vi "Power-HWP test.vi"(8 "Error In":errorcluster, 10 "Cluster In":T1={"Position"=0.0, "Is.Enabled?"=FALSE, "Is.Connected?"=FALSE, "Device SN"="55151324", "AccelerationMaximum"=10.0, "VelocityMaximum"=10.0, "Acceleration"=10.0, "Velocity"=10.0, "waitTimeout (ms)"=10000, "Model"=enum."None", "Is.Homed?"=FALSE}) -> (0 "Error Out":errorcluster)   [LabVIEW 2018]
uses:
  Hardware Mfg/Thorlabs Translation Stages/Controls/Translation Stage Cluster.ctl
  General/Controls/Translation Stage Types.ctl
  KnifeEdgeTestClt.ctl
  Hardware Mfg/Thorlabs Cage Rotation/refnum control.ctl
  General/Controls/Set Get Controls.ctl
  Hardware Mfg/Thorlabs Translation Stages/Controls/Motion Translation Module Control2.ctl
  C:/Project/SerialSectionOCT/SerialSectOCT/Labview Software/Thorlabs.MotionControl.Controls.dll
  Thorlabs.MotionControl.Controls.dll
panel:
  in  "LTS Reference":refnum<k24>(container)
  out "Power":dbl
  in  "Start":dbl
  in  "Stop":dbl
  in  "step size":dbl
  out "Wavelength [nm] 2":dbl caption="Wavelength"
  out "Avg. Time  [sec.]":dbl caption="Average Time"
  out "Average Count 2":i32 caption="Average Time"
  in  "Avg. Time (0.0) [sec.]":dbl=1.5 caption="Average Time (0.0)" min=0.1 max=5.0 step=0.1
  in  "Wavelength [nm]":dbl=840.0 caption="Wavelength (0.0)"
  in  "Average Count":i32=10 min=1 step=1
  in  "path":path=path "D:/200806 KnifeEdgeMeasurement"
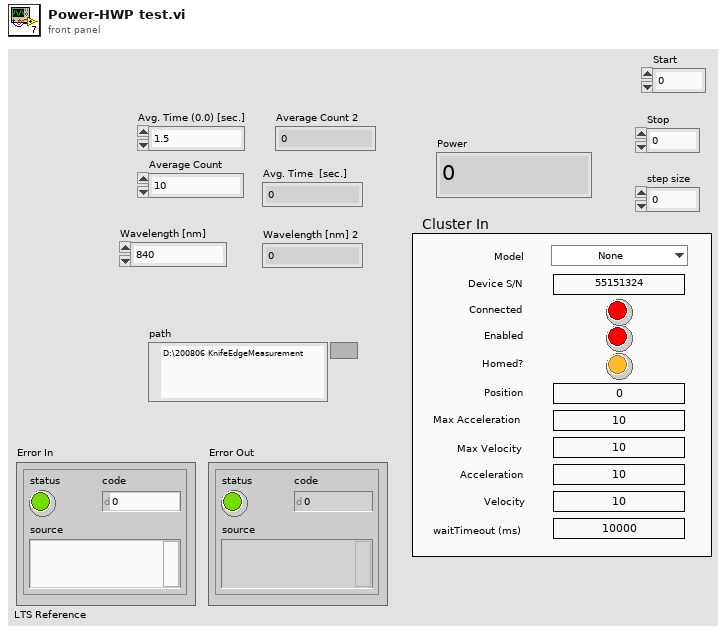
[diagram p1: front panel]
types:
  T1 = typedef "Translation Stage Cluster.ctl" = cluster{"Position":dbl, "Is.Enabled?":bool, "Is.Connected?":bool, "Device SN":string, "AccelerationMaximum":dbl, "VelocityMaximum":dbl, "Acceleration":dbl, "Velocity":dbl, "waitTimeout (ms)":i32, "Model":T2, "Is.Homed?":bool}
  T2 = typedef "Translation Stage Types.ctl" = enum16{"None", "Thorlabs LTS", "Thorlabs MLJ"}
  T3 = typedef "KnifeEdgeTestClt.ctl" = enum16{"Init Power meter", "Init Table stages", "Go stage home", "Move stage", "Measure power", "Uninit", "Generate steps"}
  T4 = typedef "refnum control.ctl" = enum16{"Get", "Init"}
  T5 = typedef "Motion Translation Module Control2.ctl" = enum16{"Init", "Home", "Status", "Velocity/Accel", "Position", "Jog", "Stop", "Uninit", "Enable", "Disable"}
  T6 = typedef "Set Get Controls.ctl" = enum16{"Set", "Get"}
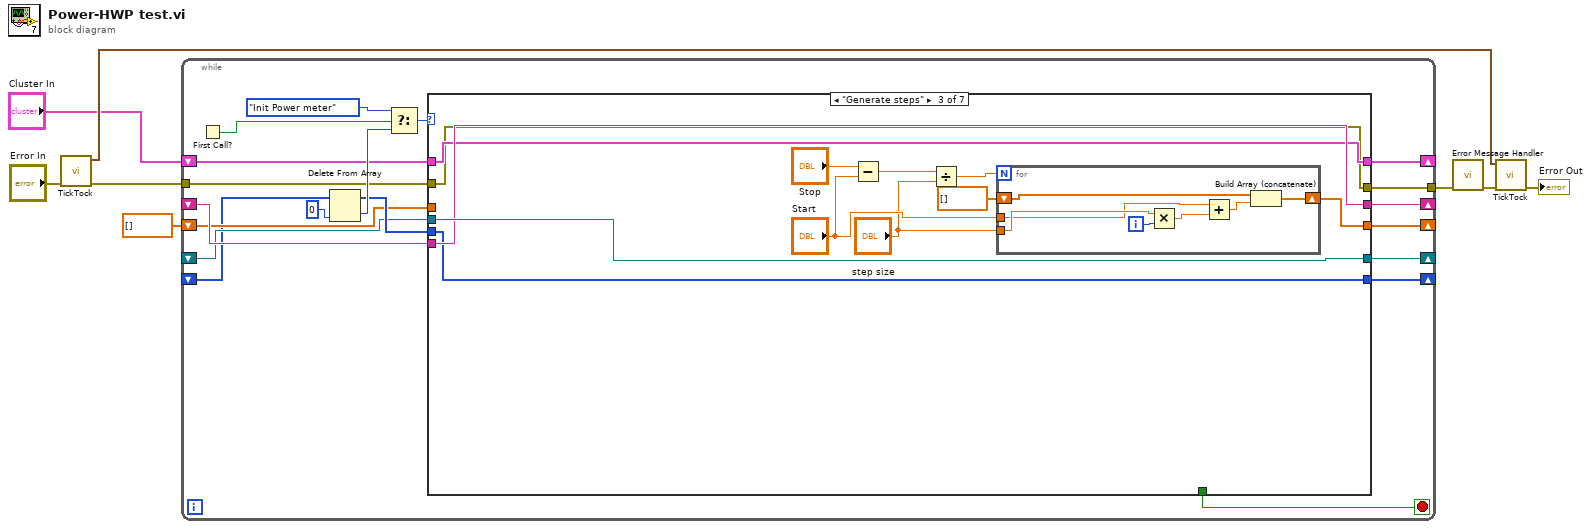
[diagram p0: block diagram]
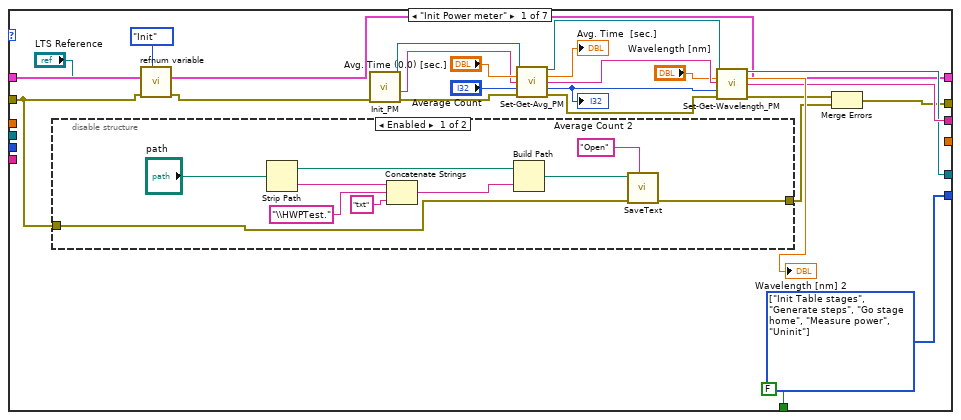
[diagram p2: hidden frame]
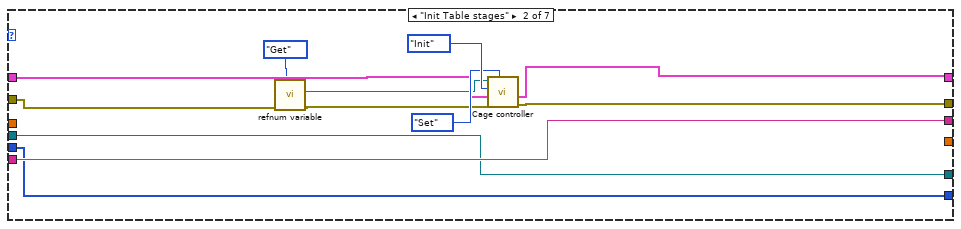
[diagram p4: hidden frame]
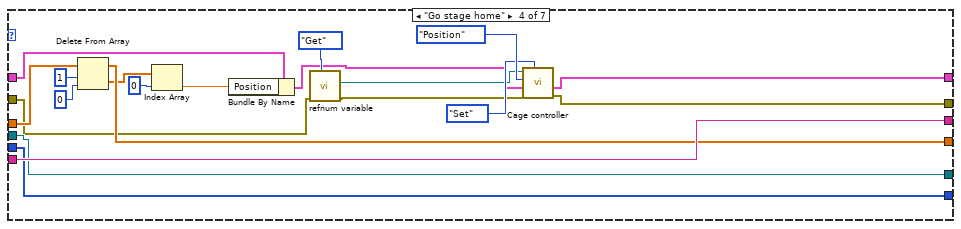
[diagram p5: hidden frame]
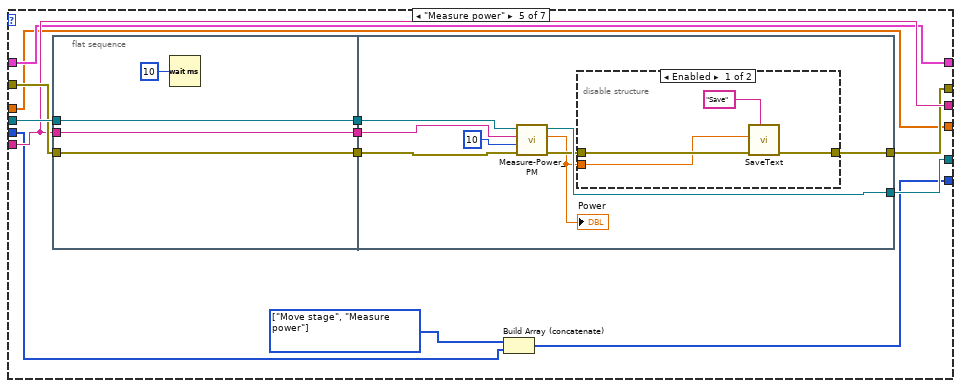
[diagram p6: hidden frame]
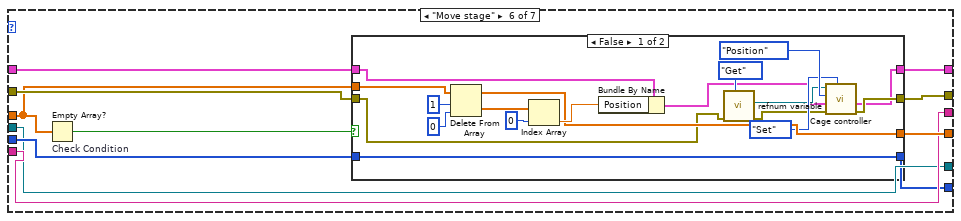
[diagram p8: hidden frame]
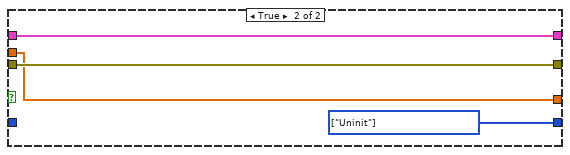
[diagram p9: hidden frame]
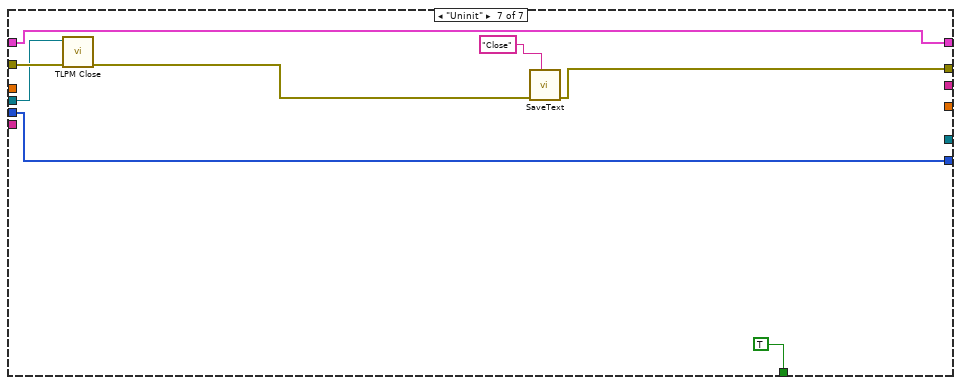
[diagram p10: hidden frame]
diagram:
  n1 = call "TickTock.vi"("Error In"="Error In") -> ("Error Out"=w6:errorcluster, "Current Time (Out)"=w4:timestamp)  [unwired: 8 in, 1 out]
  n2 = while {
    tunnel: w6 -> [w23]
    tunnel: [w22] -> w8
    shift-right: [w21] -> _
    shift-left: _ -> [w19]
    shift-right: [w20] -> _
    shift-left: _ -> [w18]
    shift-right: [w15] -> _
    shift-left: "Cluster In" -> [w16]
    shift-right: [w14] -> _
    shift-left: dbl[] [] -> [w13]
    shift-right: [w12] -> _
    shift-left: _ -> [w11]
    stop <- w10 stop-if-true
    n3 = First Call?() -> (First Call?: T/F=w9:bool)
    n4 = Delete From Array(array=w11, index=0) -> (deleted portion=w26:T3, array with subset deleted=w25:T3[])  [unwired: 1 in]
    n5 = Select(t=KnifeEdgeTestClt."Init Power meter", s=w9, f=w26) -> (s? t:f=w27:T3)
    n6 = case shown="\"Generate steps\"" w27 {
      tunnel: [w34 w71 w75 w103 w113 w144 w181] -> w12
      tunnel: w25 -> [_ w71 w75 w103 w114 w151 w181]
      tunnel: [_ _ w76 w108 w116 w153 _] -> w14
      tunnel: w23 -> [w31 w64 w82 w96 w124 w150 w183]
      tunnel: [w36 w70 w82 w95 w121 w149 w177] -> w22
      tunnel: [w39 w73 w84 w112 w122 w148 _] -> w21
      tunnel: [w38 w72 w85 w102 w123 w147 _] -> w20
      tunnel: w19 -> [_ w73 w84 w112 w122 w148 _]
      tunnel: w18 -> [_ w72 w85 w102 w125 w147 w182]
      tunnel: w16 -> [w33 w67 w83 w107 w117 w146 w180]
      tunnel: [w33 w66 w83 w93 w117 w145 w180] -> w15
      tunnel: w13 -> [_ _ _ w111 w116 w143 _]
      tunnel: [FALSE _ _ _ _ _ TRUE] -> w10
      frame "Init Power meter" {
        w34 = T3[] [enum."Init Table stages", enum."Generate steps", enum."Go stage home", enum."Measure power", enum."Uninit"] items=["Init Power meter", "Init Table stages", "Go stage home", "Move stage", "Measure power", "Uninit", "Generate steps"]
        n7 = disable-structure shown="Enabled" {
          disable-tunnel: w31 -> [w56 _]
          disable-tunnel: [w55 _] -> w37
          frame Enabled {
            n8 = Strip Path(path="path") -> (stripped path=w53:path, name=w59:string)
            n9 = Concatenate Strings(w59, "\\HWPTest." ("string"), "txt" ("string")) -> (w54:string)
            n10 = Build Path(base path=w53, name or relative path=w54) -> (appended path=w52:path)
            n11 = call "SaveText.vi"("action"="Open", "error in"=w56, "file path (use dialog)"=w52) -> ("error out"=w55:errorcluster)  [unwired: 8 in]
          }
          frame Disabled {
          }
        }
        n12 = call "refnum variable.vi"("action"=refnum_control."Init", "error in (no error)"=w31, "reference in"="LTS Reference") -> ("error out"=w30:errorcluster)  [unwired: 7 in, 1 out]
        n13 = call "Init_PM.vi"("error in (no error)"=w30) -> ("error out"=w40:errorcluster, "Sensor Name"=w41:string, "instrument handle out"=w42:refnum<visa-resource-name>)  [unwired: 8 in]
        n14 = call "Set-Get-Avg_PM.vi"("instrument handle"=w42, "Average Time (0.0)"="Avg. Time (0.0) [sec.]", "Sensor"=w41, "Average Count"="Average Count", "error in (no error)"=w40) -> ("instrument handle out"=w49:refnum<visa-resource-name>, "Average Time"=→"Avg. Time  [sec.]":dbl, "Sensor 2"=w47:string, "Average Count"=w46:i32, "error out"=w50:errorcluster)  [unwired: 6 in]
        "Average Count 2" <- w46
        n15 = call "Set-Get-Wavelength_PM.vi"("instrument handle"=w49, "Wavelength"="Wavelength [nm]", "Sensor Name"=w47, "Average Count"=w46, "error in (no error)"=w50) -> ("instrument handle out"=w38:refnum<visa-resource-name>, "Wavelength"=→"Wavelength [nm] 2":dbl, "Sensor Name 2"=w39:string, "error out"=w35:errorcluster)  [unwired: 6 in, 1 out]
        n16 = Merge Errors(w35, w37) -> (w36:errorcluster)
      }
      frame "Init Table stages" {
        n17 = call "refnum variable.vi"("action"=refnum_control."Get", "error in (no error)"=w64) -> ("error out"=w63:errorcluster, "reference in 2"=w62:refnum<k24>)  [unwired: 8 in]
        n18 = call "Cage controller.vi"("Set/Get"=Set_Get_Controls."Set", "error in (no error)"=w63, "Cluster In"=w67, "Action"=Motion_Translation_Module_Control2."Init", "reference in"=w62) -> ("error out"=w70:errorcluster, "Cluster out"=w66:T1)  [unwired: 4 in, 1 out]
      }
      frame "Generate steps" {
        n19 = Subtract(x="Stop", y="Start") -> (x-y=w80:dbl)
        n20 = Divide(x=w80, y="step size") -> (x/y=w79:dbl)
        n21 = for {
          N: w79 -> [_]
          tunnel: "Start" -> [w90]
          tunnel: "step size" -> [w91]
          shift-right: [w87] -> w76
          shift-left: dbl[] [] -> [w86]
          i -> [w92]
          n22 = Multiply(x=w91, y=w92) -> (x*y=w89:dbl)
          n23 = Add(x=w90, y=w89) -> (x+y=w88:dbl)
          n24 = Build Array (concatenate)(w86, w88) -> (w87:dbl[])
        }
      }
      frame "Go stage home" {
        n25 = Delete From Array(array=w111, length=1, index=0) -> (deleted portion=w106:dbl[], array with subset deleted=w108:dbl[])
        n26 = Index Array(array=w106, index=0) -> (element=w104:dbl)
        n27 = Bundle By Name(cluster=w107, "Position"=w104) -> (w94:T1)
        n28 = call "refnum variable.vi"("action"=refnum_control."Get", "error in (no error)"=w96) -> ("error out"=w98:errorcluster, "reference in 2"=w97:refnum<k24>)  [unwired: 8 in]
        n29 = call "Cage controller.vi"("Set/Get"=Set_Get_Controls."Set", "error in (no error)"=w98, "Cluster In"=w94, "Action"=Motion_Translation_Module_Control2."Position", "reference in"=w97) -> ("error out"=w95:errorcluster, "Cluster out"=w93:T1)  [unwired: 4 in, 1 out]
      }
      frame "Measure power" {
        w115 = T3[] [enum."Move stage", enum."Measure power"] items=["Init Power meter", "Init Table stages", "Go stage home", "Move stage", "Measure power", "Uninit", "Generate steps"] ("element")
        n30 = flat-sequence {
          tunnel: w122 -> [w127]
          tunnel: w124 -> [w128]
          tunnel: w125 -> [w129]
          tunnel: [w129] -> w120
          tunnel: [w128] -> w119
          tunnel: [w127] -> w118
          tunnel: [w135] -> w123
          tunnel: [w133] -> w121
          tunnel: w120 -> [w137]
          tunnel: w119 -> [w136]
          tunnel: w118 -> [w134]
          frame #0 {
            n31 = Wait (ms)(milliseconds to wait=u32 10) -> ()  [unwired: 1 out]
          }
          frame #1 {
            n32 = call "Measure-Power_PM.vi"("error in (no error)"=w136, "Numeric"=10, "Sensor"=w134, "instrument handle"=w137) -> ("error out"=w131:errorcluster, "Power"=w130:dbl, "instrument handle out"=w135:refnum<visa-resource-name>)  [unwired: 5 in]
            "Power" <- w130
            n33 = disable-structure shown="Enabled" {
              disable-tunnel: [w141 w142] -> w133
              disable-tunnel: w131 -> [w140 w142]
              disable-tunnel: w130 -> [w138 _]
              frame Enabled {
                n34 = call "SaveText.vi"("action"="Save", "error in"=w140, "data in"=w138) -> ("error out"=w141:errorcluster)  [unwired: 8 in]
              }
              frame Disabled {
              }
            }
          }
        }
        n35 = Build Array (concatenate)(w115, w114) -> (w113:T3[])
      }
      frame "Move stage" {
        n36 = Empty Array? "Check Condition"(array=w143) -> (empty?=w152:bool)
        n37 = case shown="False" w152 {
          tunnel: [w164 w174] -> w153
          tunnel: w151 -> [w163 _]
          tunnel: [w163 w172] -> w144
          tunnel: w150 -> [w157 w175]
          tunnel: [w156 w175] -> w149
          tunnel: w146 -> [w166 w173]
          tunnel: [w155 w173] -> w145
          tunnel: w143 -> [w165 w174]
          frame False {
            n38 = Delete From Array(array=w165, length=1, index=0) -> (deleted portion=w169:dbl[], array with subset deleted=w164:dbl[])
            n39 = Index Array(array=w169, index=0) -> (element=w167:dbl)
            n40 = Bundle By Name(cluster=w166, "Position"=w167) -> (w154:T1)
            n41 = call "refnum variable.vi"("action"=refnum_control."Get", "error in (no error)"=w157) -> ("error out"=w159:errorcluster, "reference in 2"=w158:refnum<k24>)  [unwired: 8 in]
            n42 = call "Cage controller.vi"("Set/Get"=Set_Get_Controls."Set", "error in (no error)"=w159, "Cluster In"=w154, "Action"=Motion_Translation_Module_Control2."Position", "reference in"=w158) -> ("error out"=w156:errorcluster, "Cluster out"=w155:T1)  [unwired: 4 in, 1 out]
          }
          frame True {
            w172 = T3[] [enum."Uninit"] items=["Init Power meter", "Init Table stages", "Go stage home", "Move stage", "Measure power", "Uninit", "Generate steps"]
          }
        }
      }
      frame "Uninit" {
        n43 = call "TLPM Close.vi"("error in (no error)"=w183, "instrument handle"=w182) -> ("error out"=w178:errorcluster)  [unwired: 9 in]
        n44 = call "SaveText.vi"("action"="Close", "error in"=w178) -> ("error out"=w177:errorcluster)  [unwired: 9 in]
      }
    }
  }
  n45 = call "Error Message Handler.vi"("Error In"=w8) -> ("Error Out"=w3:errorcluster)  [unwired: 9 in, 1 out]
  n46 = call "TickTock.vi"("Error In"=w3, "Current Time (In)"=w4) -> ("Error Out"=→"Error Out":errorcluster)  [unwired: 7 in, 2 out]
